vi "Test FTP 2.vi"() -> ()   [LabVIEW 2012]
uses:
  <vilib>/FTP/NI_FTP.lvlib
panel:
  out "error out 2":errorcluster
  out "file error":errorcluster
  out "code":i32
  out "sub class":u16(ring) items=["Syntax", "Information", "Connection", "Authentication", "Unspecified", "File System", "unknown"]
  out "class":T1(ring)=enum."500 - Permanent"
  out "error out":errorcluster
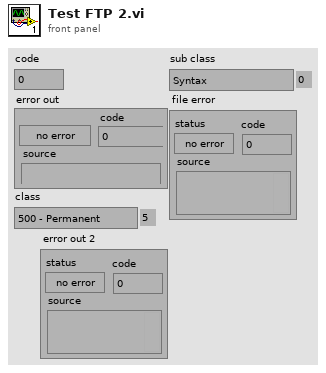
[diagram p1: front panel]
types:
  T1 = enum16{"unknown", "100 + Prelim", "200 + ", "300 + Intermed", "400 - Transient", "500 - Permanent"}
  T2 = typedef "NI_FTP.lvlib/FTP Session.ctl" = refnum<k5>
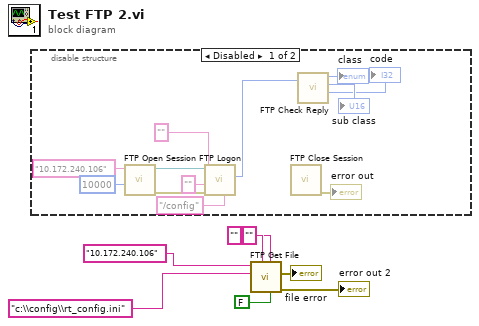
[diagram p0: block diagram]
diagram:
  n1 = disable-structure shown="Disabled" {
    frame Disabled {
      n2 = call <vilib>:"FTP Open Session.vi"("timeout ms (60000)"=10000, "address"="10.172.240.106") -> ("error out"=w15:errorcluster, "ftp session"=w16:T2)  [unwired: 6 in, 2 out]
      n3 = call <vilib>:"FTP Logon.vi"("starting path"="/config", "error in (no error)"=w15, "password"="", "user"="", "ftp session"=w16) -> ("reply code"=w12:i32)  [unwired: 3 in, 3 out]
      n4 = call <vilib>:"FTP Close Session.vi"() -> ("error out"=→"error out":errorcluster)  [unwired: 8 in, 3 out]
      n5 = call <vilib>:"FTP Check Reply.vi"("reply"=w12) -> ("class"=→"class":T1, "sub class"=→"sub class":u16, "code"=→"code":i32)  [unwired: 1 in, 1 out]
    }
    frame Enabled {
    }
  }
  n6 = call <vilib>:"FTP Get File.vi"("active (T)"=FALSE, "password"="", "user"="", "remote path"="c:\\config\\rt_config.ini", "host"="10.172.240.106" ("address")) -> ("error out"=→"error out 2":errorcluster, "file error"=→"file error":errorcluster)  [unwired: 5 in]
